vi "fpga_Tick Node.vi"() -> (3 "millisecond timer value":u32)   [LabVIEW 2012, in "NI_EP_Protection_FPGA.lvlib"]
uses:
  <vilib>/addons/Electrical Power/Protection/NI_EP_Protection_FPGA.lvlib
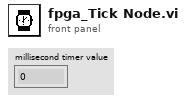
[diagram p1: front panel]
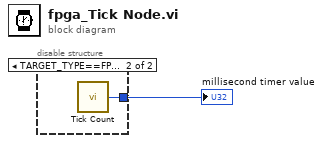
[diagram p0: block diagram]
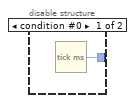
[diagram p2: hidden frame]
diagram:
  n1 = disable-structure shown="TARGET_TYPE==FPGA" {
    disable-tunnel: [w2 w3] -> w1
    frame condition #0 {
      n2 = Tick Count (ms)() -> (millisecond timer value=w2:u32)
    }
    frame condition #1 (active) {
      n3 = call "Tick Count"() -> ("Tick Count(mSec)"=w3:u32)
    }
  }
  "millisecond timer value" <- w1
